vi "Read Sorting Enabled.vi"(8 "error in":errorcluster, 11 "EngineTags in":refnum<class "Engine Mappings.lvclass">) -> (0 "error out":errorcluster, 2 "sort type":T1, 3 "EngineTags out":refnum<class "Engine Mappings.lvclass">)   [LabVIEW 2013, in "PL Framework Configuration Tool.lvlib" / "Engine Mappings.lvclass"]
uses:
  Engine Mappings.lvclass
  mapping sort type.ctl
  Engine Mappings.lvclass/Engine Mappings.ctl
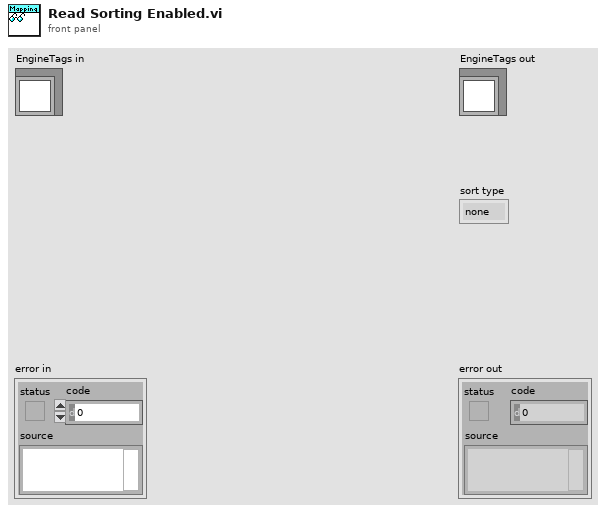
[diagram p1: front panel]
types:
  T1 = typedef "PL Framework Configuration Tool.lvlib/Engine Mappings.lvclass/mapping sort type.ctl" = enum16{"none", "asc", "desc"}
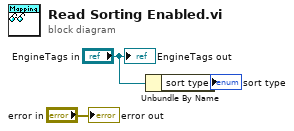
[diagram p0: block diagram]
diagram:
  n1 = Unbundle By Name("EngineTags in") -> ("sort type"=→"sort type":T1)
  "error out" <- "error in"
  "EngineTags out" <- "EngineTags in"
